vi "Add Credentials.vi"(8 "error in (no error)":errorcluster, 10 "Credentials":refnum<k24>, 11 "WebProxy_NET in":refnum<class "WebProxy_NET.lvclass">) -> (0 "error out":errorcluster, 3 "WebProxy_NET out":refnum<class "WebProxy_NET.lvclass">)   [LabVIEW 2018, in "HttpClient_NET.lvlib" / "WebProxy_NET.lvclass"]
doc: "<b> </b> <b> </b>\nHttpClient_NET\nJustin Young - Viviota\nCopyright (c) 2021\nLicense: BSD"
uses:
  WebProxy_NET.lvclass
  WebProxy_NET.lvclass/WebProxy_NET.ctl
  Accessors/Read NET_WebProxy.vi
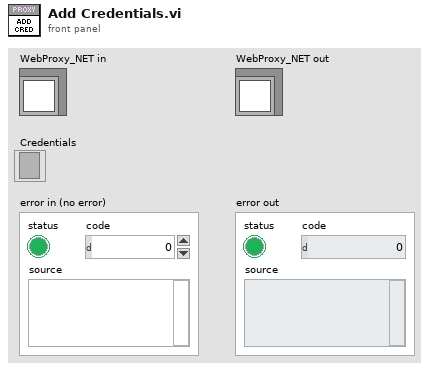
[diagram p1: front panel]
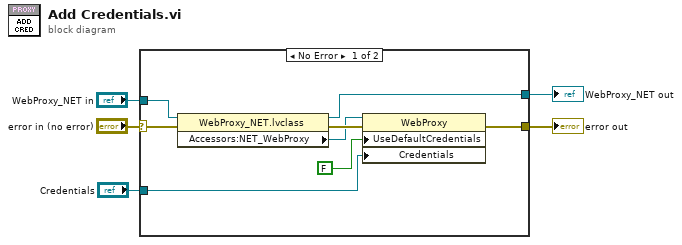
[diagram p0: block diagram]
diagram:
  n1 = case shown="No Error" "error in (no error)" {
    selector: "error in (no error)" -> [w11 w14]
    tunnel: [w13 w14] -> w5
    tunnel: [w8 w15] -> w3
    tunnel: "WebProxy_NET in" -> [w7 w15]
    tunnel: "Credentials" -> [w6 _]
    frame No Error {
      n2 = property class="WebProxy_NET.lvclass"(reference=w7, error in=w11) -> (reference out=w8:refnum<class "WebProxy_NET.lvclass">, error out=w12:errorcluster, "Accessors:NET_WebProxy"=w9:refnum<k24>)
      n3 = property class="WebProxy"(reference=w9, error in=w12, "UseDefaultCredentials"=FALSE, "Credentials"=w6) -> (error out=w13:errorcluster)  [unwired: 1 out]
    }
    frame Error {
    }
  }
  "error out" <- w5
  "WebProxy_NET out" <- w3
